vi "Setup ramp in awg.vi"(4 "Channel Name (1)":u16(ring)=1 items=["1"=1, "2"=2, "3"=3, "4"=4], 5 "VISA resource name":refnum<visa-resource-name>="GPIB0::1::INSTR", 7 "End time S":dbl=0.00015, 8 "error in (no error)":errorcluster, 9 "Ramp time S":dbl=0.01, 10 "Delay time S":dbl=0.01, 11 "Sampling Frequency (Hz)":u64=10000000) -> (0 "error out":errorcluster)   [LabVIEW 2021]
uses:
  <vilib>/Waveform/DWDTOps.llb/DWDT Boolean Array to Digital.vi
  <instrlib>/Tektronix AWG 5000 7000 Series/Public/Configure/Channel/Assign Output Waveform (From Waveform List).vi
  <instrlib>/Tektronix AWG 5000 7000 Series/Public/Configure/Configure Output Timing (Sampling Frequency).vi
  <instrlib>/Tektronix AWG 5000 7000 Series/Tektronix AWG 5000 7000 Series.lvlib
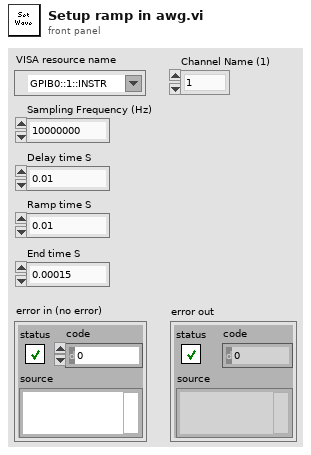
[diagram p1: front panel]
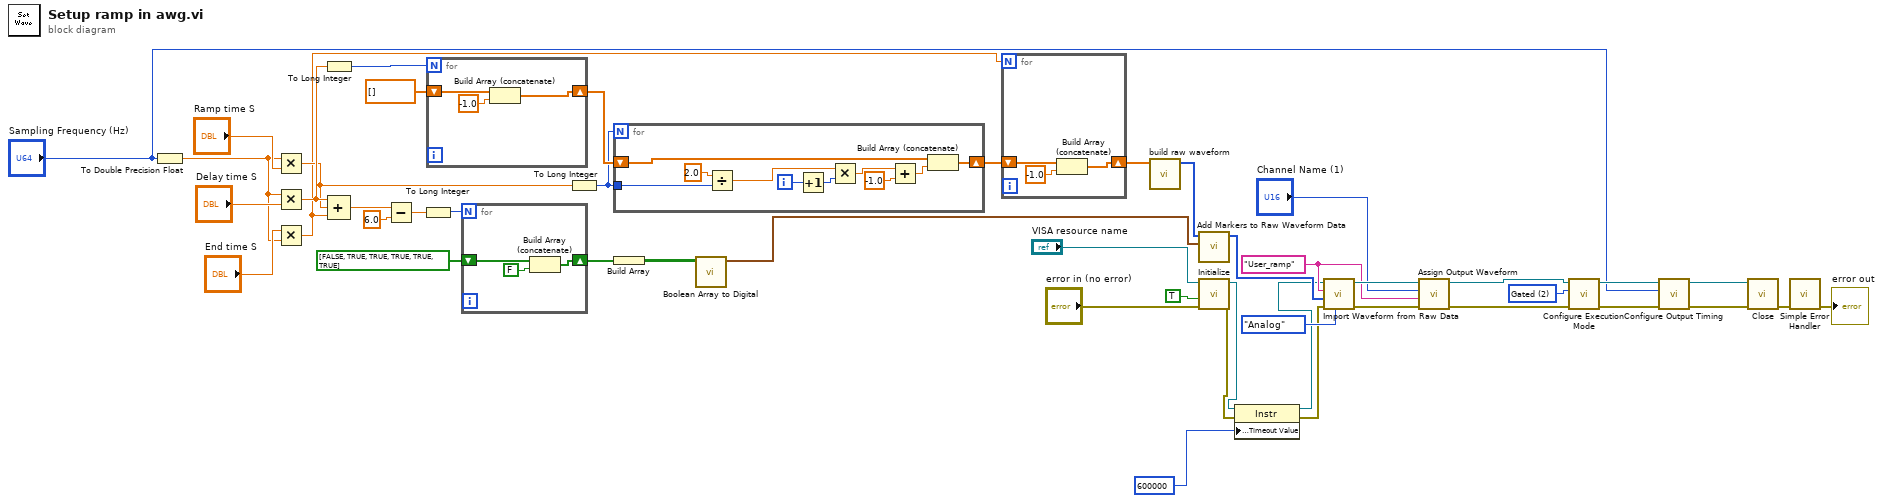
[diagram p0: block diagram]
diagram:
  w15 = u16 2 items=["Continuous", "Triggered", "Gated", "Sequence", "Triggered Continuous"] ("Execution Mode (0 : Continuous)")
  w17 = "User_ramp" ("Waveform Name")
  n1 = To Double Precision Float(number="Sampling Frequency (Hz)") -> (double precision float=w12:dbl)
  n2 = Multiply(x=w12, y="Ramp time S") -> (x*y=w26:dbl)
  n3 = Multiply(x=w12, y="Delay time S") -> (x*y=w27:dbl)
  n4 = Multiply(x="End time S", y=w12) -> (x*y=w25:dbl)
  n5 = To Long Integer(number=w27) -> (32bit integer=w10:i32)
  n6 = Compound Arithmetic op=ADD(w27, w26, w25) -> (w24:dbl)
  n7 = Subtract(x=w24, y=6.0) -> (x-y=w22:dbl)
  n8 = To Long Integer(number=w22) -> (32bit integer=w11:i32)
  n9 = for {
    N: w10 -> [_]
    shift-right: [w48] -> w34
    shift-left: dbl[] [] -> [w49]
    n10 = Build Array (concatenate)(w49, -1.0) -> (w48:dbl[])
  }
  n11 = for {
    N: w11 -> [_]
    shift-right: [w50] -> w21
    shift-left: bool[] [FALSE, TRUE, TRUE, TRUE, TRUE, TRUE] -> [w52]
    n12 = Build Array (concatenate)(w52, FALSE) -> (w50:bool[])
  }
  n13 = To Long Integer(number=w26) -> (32bit integer=w9:i32)
  n14 = for {
    N: w9 -> [_]
    tunnel: w9 -> [w61]
    shift-right: [w53] -> w33
    shift-left: w34 -> [w55]
    i -> [w59]
    n15 = Divide(x=2.0, y=w61) -> (x/y=w60:dbl)
    n16 = Increment(x=w59) -> (x+1=w58:i32)
    n17 = Multiply(x=w60, y=w58) -> (x*y=w57:dbl)
    n18 = Add(x=w57, y=-1.0) -> (x+y=w54:dbl)
    n19 = Build Array (concatenate)(w55, w54) -> (w53:dbl[])
  }
  n20 = Build Array(w21) -> (w20:bool[][])
  n21 = call-poly <vilib>:"Boolean Array to Digital.vi"("boolean array"=w20) -> ("digital waveform"=w7:digitalwaveform)  [unwired: 9 in, 1 out]
  n22 = for {
    N: w25 -> [_]
    shift-right: [w64] -> w29
    shift-left: w33 -> [w65]
    n23 = Build Array (concatenate)(w65, -1.0) -> (w64:dbl[])
  }
  n24 = call "build raw waveform.vi"("Y"=w29) -> ("Raw Waveform Data"=w8:u8[])  [unwired: 10 in]
  n25 = call <instrlib>:"Add Markers to Raw Waveform Data.vi"("Markers"=w7, "Raw Waveform Data"=w8) -> ("Raw Waveform Data with Markers"=w6:u8[])  [unwired: 9 in]
  n26 = call <instrlib>:"Initialize.vi"("error in (no error)"="error in (no error)", "Reset (False)"=TRUE ("Reset? (F: No)"), "VISA resource name"="VISA resource name") -> ("error out"=w2:errorcluster, "VISA resource name out"=w4:refnum<visa-resource-name>)  [unwired: 7 in]
  n27 = property class="Instr"(reference=w4, error in=w2, "General Settings:Timeout Value"=u32 600000) -> (reference out=w3:refnum<visa-resource-name>, error out=w1:errorcluster)
  n28 = call <instrlib>:"Import Waveform from Raw Data.vi"("Representation (1 : Analog)"=enum16{"Integer", "Analog"}."Analog", "error in (no error)"=w1, "Raw Data"=w6, "Waveform Name"=w17, "VISA resource name"=w3) -> ("error out"=w16:errorcluster, "VISA resource name out"=w18:refnum<visa-resource-name>)  [unwired: 5 in]
  n29 = call-poly <instrlib>:"Assign Output Waveform.vi"("error in (no error)"=w16, "Waveform"=w17, "Channel Name (1)"="Channel Name (1)", "VISA resource name"=w18) -> ("error out"=w44:errorcluster, "VISA resource name out"=w45:refnum<visa-resource-name>)  [unwired: 6 in]
  n30 = call <instrlib>:"Configure Execution Mode.vi"("error in (no error)"=w44, "Execution Mode (0 : Continuous)"=w15, "VISA resource name"=w45) -> ("error out"=w42:errorcluster, "VISA resource name out"=w43:refnum<visa-resource-name>)  [unwired: 7 in]
  n31 = call-poly <instrlib>:"Configure Output Timing.vi"("error in (no error)"=w42, "Sampling Frequency (Hz) (100MHz)"="Sampling Frequency (Hz)", "VISA resource name"=w43) -> ("error out"=w40:errorcluster, "VISA resource name out"=w41:refnum<visa-resource-name>)  [unwired: 7 in]
  n32 = call <instrlib>:"Close.vi"("error in (no error)"=w40, "VISA resource name"=w41) -> ("error out"=w39:errorcluster)  [unwired: 9 in]
  n33 = call <vilib>:"Simple Error Handler.vi"("error in (no error)"=w39) -> ("error out"=→"error out":errorcluster)  [unwired: 4 in, 4 out]
